vi "Read Write TimeStamp.vi"(11 "Error in":errorcluster, 13 "Enum":enum16{"Read Time", "Write Time"}(ring)=enum."Write Time") -> (2 "isEmpty?":bool, 4 "Error?":bool, 6 "Time Stamp":timestamp, 15 "Error out":errorcluster)   [LabVIEW 2022 SP3]
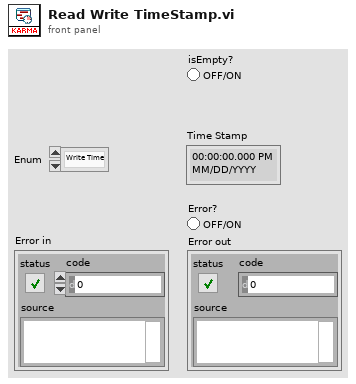
[diagram p1: front panel]
types:
  T1 = enum16{"open", "replace", "create", "open or create", "replace or create", "replace or create with confirmation"}
  T2 = typedef "Paths.ctl" = cluster{"Configuration":path, "Event Logs":path, "Error Logs":path, "Configuration.ini":path}
  T3 = typedef "LVDateTimeRec.ctl" = cluster{"fractional second":dbl, "second":i32, "minute":i32, "hour":i32, "day of month":i32, "month":i32, "year":i32, "day of week":i32, "day of year":i32, "DST":i32}
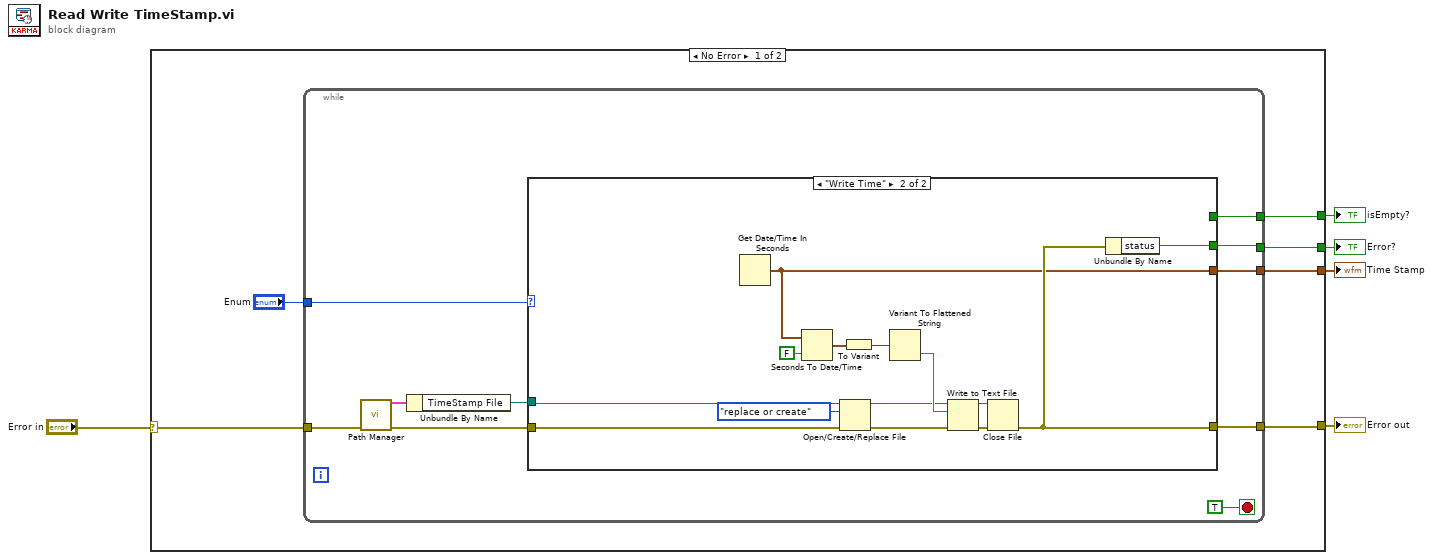
[diagram p0: block diagram]
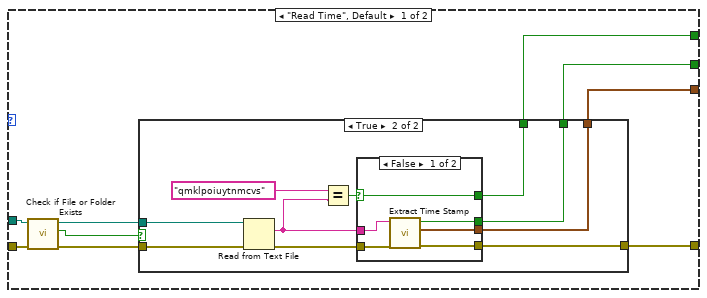
[diagram p2: hidden frame]
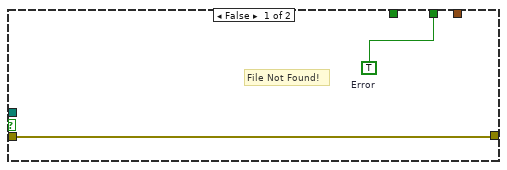
[diagram p3: hidden frame]
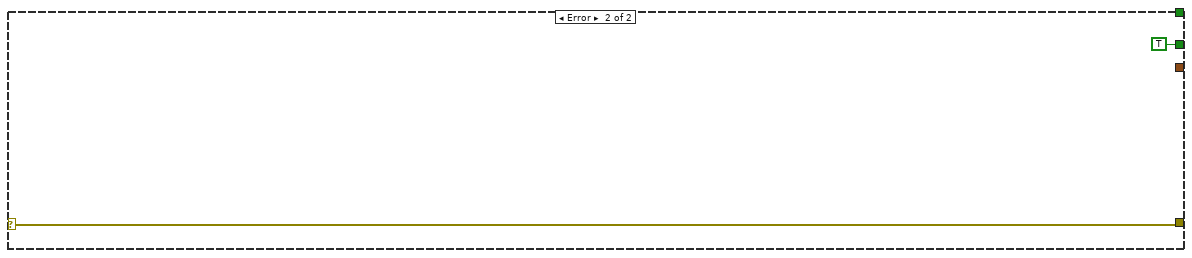
[diagram p5: hidden frame]
diagram:
  n1 = case shown="No Error" "Error in" {
    selector: "Error in" -> [w10 w65]
    tunnel: [w9 TRUE ("status")] -> w4
    tunnel: [w8 _] -> w3
    tunnel: [w7 w65] -> w2
    tunnel: [w6 _] -> w1
    frame No Error {
      n2 = while {
        tunnel: "Enum" -> [w21]
        tunnel: w10 -> [w19]
        tunnel: [w15] -> w9
        tunnel: [w14] -> w8
        tunnel: [w13] -> w7
        tunnel: [w12] -> w6
        stop <- TRUE stop-if-true
        n3 = call "Path Manager.vi"("error in (no error)"=w19) -> ("Cluster"=w17:T2, "Error out"=w18:errorcluster)  [unwired: 13 in]
        n4 = Unbundle By Name(w17) -> ("TimeStamp File"=w16:path)
        n5 = case shown="\"Write Time\"" w21 {
          tunnel: w18 -> [w27 w62]
          tunnel: w16 -> [w24 w61]
          tunnel: [w30 w55] -> w15
          tunnel: [w29 w54] -> w14
          tunnel: [w28 w56] -> w13
          tunnel: [w22 _] -> w12
          frame "Read Time", Default {
            n6 = call <vilib>:"Check if File or Folder Exists.vi"("error in (no error)"=w27, "path"=w24) -> ("error out"=w26:errorcluster, "file or folder exists?"=w25:bool, "dup path"=w23:path)  [unwired: 7 in]
            n7 = case shown="True" w25 {
              tunnel: w26 -> [w32 w42]
              tunnel: w23 -> [_ w41]
              tunnel: [w31 w39] -> w30
              tunnel: [_ w38] -> w29
              tunnel: [w32 w37] -> w28
              tunnel: [_ w36] -> w22
              frame False {
                w31 = TRUE  # Error
                # "File Not Found!"
              }
              frame True {
                n8 = Read from Text File(file (use dialog)=w41, error in=w42) -> (text=w34:string, error out=w40:errorcluster)  [unwired: 2 in, 2 out]
                n9 = Equal?(x="qmklpoiuytnmcvs", y=w34) -> (x = y?=w35:bool)
                n10 = case shown="False" w35 {
                  selector: w35 -> [w43 w49]
                  tunnel: w40 -> [w48 w50]
                  tunnel: [w47 _] -> w39
                  tunnel: [w46 _] -> w38
                  tunnel: [w45 w50] -> w37
                  tunnel: w34 -> [w44 _]
                  tunnel: [w43 w49] -> w36
                  frame False {
                    n11 = call "Extract Time Stamp.vi"("Error in"=w48, "String"=w44) -> ("Error out"=w45:errorcluster, "Time Stamp"=w46:timestamp, "Error"=w47:bool)  [unwired: 7 in]
                  }
                  frame True {
                  }
                }
              }
            }
          }
          frame "Write Time" {
            n12 = Get Date/Time In Seconds() -> (seconds since 1Jan1904=w54:timestamp)
            n13 = Seconds To Date/Time(time stamp (now)=w54, to UTC (F)=FALSE) -> (date time rec=w52:T3)
            n14 = Open/Create/Replace File(file path (use dialog)=w61, operation (0:open)=T1."replace or create") -> (refnum out=w59:refnum<file>)  [unwired: 4 in, 2 out]
            n15 = To Variant(anything=w52) -> (Variant=w51:variant)
            n16 = Variant To Flattened String(Variant=w51) -> (data string=w63:string)  [unwired: 1 out]
            n17 = Write to Text File(file (use dialog)=w59, text=w63, error in=w62) -> (refnum out=w58:refnum<file>, error out=w57:errorcluster)  [unwired: 1 in, 1 out]
            n18 = Close File(refnum=w58, error in=w57) -> (error out=w56:errorcluster)  [unwired: 1 out]
            n19 = Unbundle By Name(w56) -> ("status"=w55:bool)
          }
        }
      }
    }
    frame Error {
    }
  }
  "Error?" <- w4
  "Time Stamp" <- w3
  "Error out" <- w2
  "isEmpty?" <- w1
